vi "test_ImageAssemblerMG090623Binning.vi"() -> ()   [LabVIEW 2010, in "ImageAssemblerMG090623Binning.lvclass"]
uses:
  ImageAssemblerMG090623Binning.lvclass
  main/labview_source/type_definitions/clusters/controls_refs.ctl
  <vilib>/vision/Image Controls.llb/IMAQ Image.ctl
  common/classes/Image/Image/Image.lvclass
  GenericImageAssembler/GenericImageAssembler/trigger_enum.ctl
  ImageAssemblerMG090623Binning.lvclass/ImageAssemblerMG090623Binning.ctl
  GenericImageAssembler/GenericImageAssembler/GenericImageAssembler.lvclass
panel:
  in  "frame rate for sending":dbl[unit]=20.0
  in  "frame rate":dbl[unit]=1.0
  in  "number of images to send":i32=2
  out "loop counter":i32
  in  "send continuously button":bool
  in  "start button":bool
  in  "y resolution":i32=100
  out "input image array":T1[](array[plugin-control])
  in  "stop":bool
  in  "x resolution":i32=100
  in  "number of channels":i32=1 min=1
  in  "send  button":bool
  in  "load button":bool
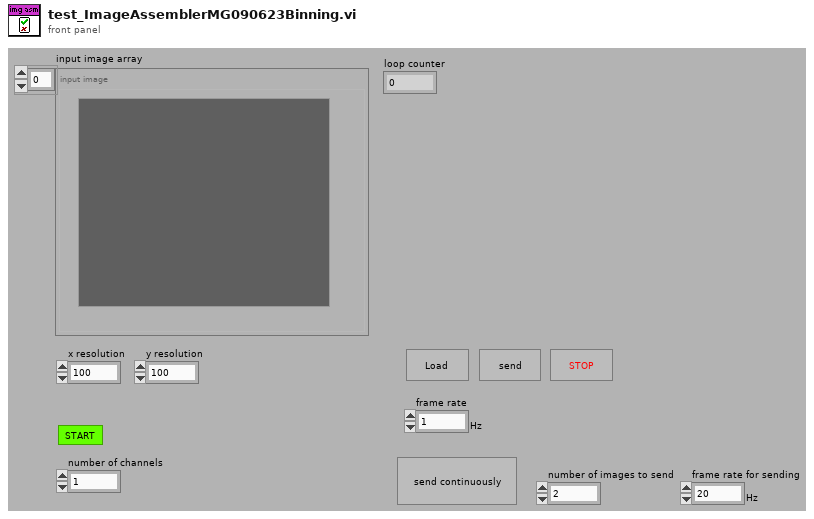
[diagram p1: front panel]
types:
  T1 = typedef "IMAQ Image.ctl" = refnum<image>
  T2 = typedef "Image Type" = u32
  T3 = typedef "controls_refs.ctl" = cluster{"scan start button":refnum<vi>, "tabs":cluster{"main":refnum<vi>, "settings":refnum<vi>}, "subpanels":cluster{"imagingMode":refnum<vi>, "scanHead":refnum<vi>, "display":refnum<vi>, "experimentController":refnum<vi>, "instrument":refnum<vi>, "stage":refnum<vi>, "stimulator":refnum<vi>, "dataCollection":refnum<vi>, "analyser":refnum<vi>, "daq":refnum<vi>, "imageAssembler":refnum<vi>}, "drop-downs":cluster{"run mode":refnum<vi>, "imagingMode":refnum<vi>, "experimentalController":refnum<vi>, "objective":refnum<vi>}, "status lights":cluster{"experimentController":refnum<vi>, "imagingMode":refnum<vi>, "scanHead":refnum<vi>, "daq":refnum<vi>, "imageAssembler":refnum<vi>, "dataCollection":refnum<vi>, "display":refnum<vi>, "analyser":refnum<vi>, "stage":refnum<vi>, "stimulator":refnum<vi>, "instrument":refnum<vi>}, "message":refnum<vi>, "stimulator enabled?":refnum<vi>, "saving":cluster{"data folder path":refnum<vi>, "file base name":refnum<vi>, "notebook":refnum<vi>}, "progress bar":refnum<vi>, "update icon":refnum<vi>, "title":refnum<vi>, "main vi":refnum<vi>, "user":refnum<vi>, "exit_button":refnum<vi>, "CPU usage %":refnum<vi>}
  T4 = typedef "GenericImageAssembler.lvclass/trigger_enum.ctl" = enum16{"NULL", "start", "stop"}
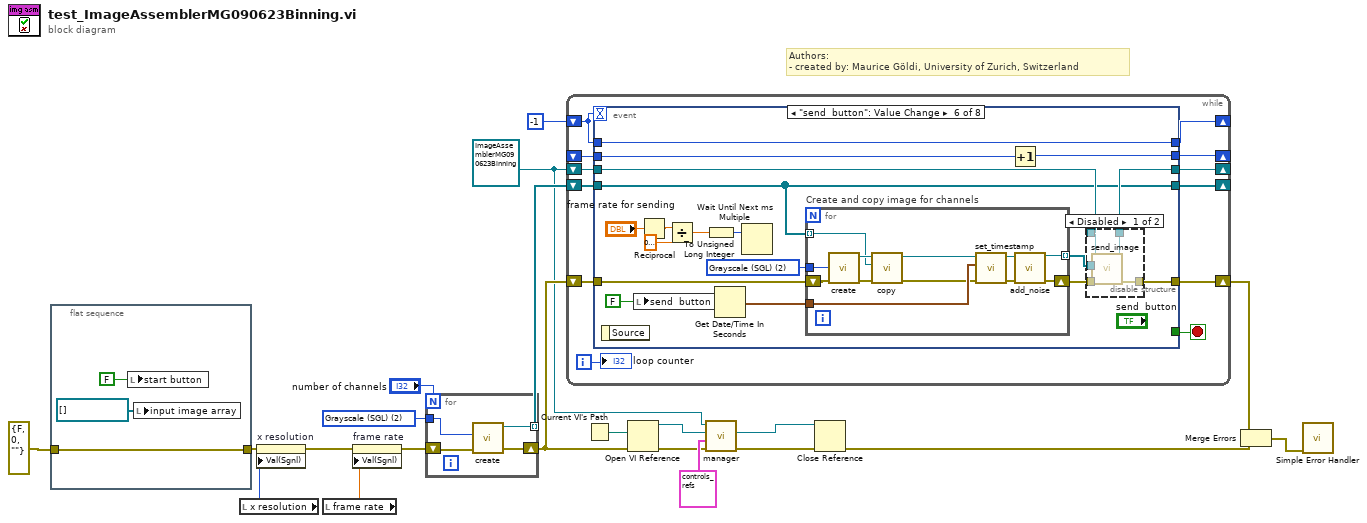
[diagram p0: block diagram]
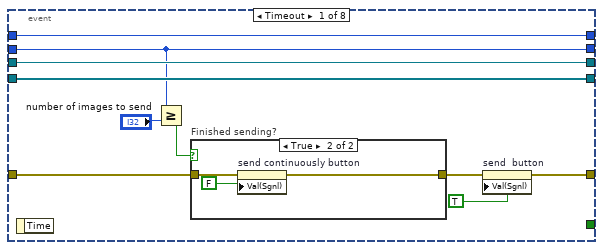
[diagram p2: hidden frame]
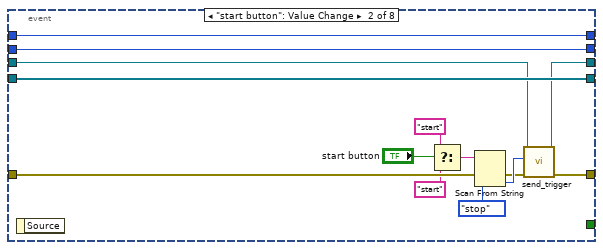
[diagram p4: hidden frame]
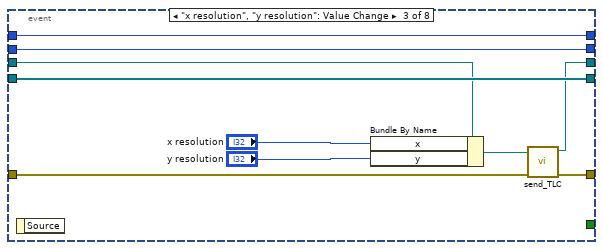
[diagram p5: hidden frame]
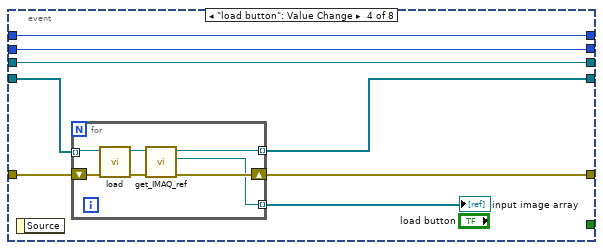
[diagram p6: hidden frame]
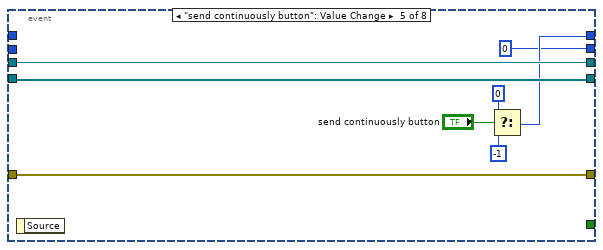
[diagram p7: hidden frame]
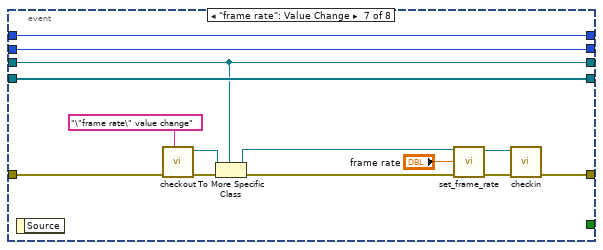
[diagram p9: hidden frame]
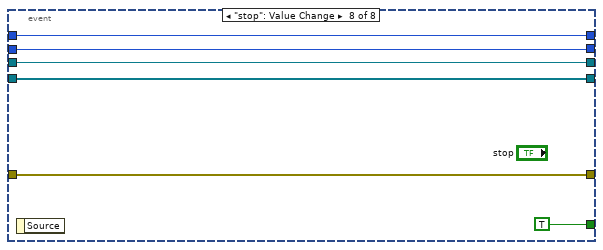
[diagram p10: hidden frame]
diagram:
  w1 = refnum<class "ImageAssemblerMG090623Binning.lvclass"> refnum ("MG090623BinningImageAssembler.lvclass")
  w13 = T2 2 items=["Grayscale (U8)", "Grayscale (I16)", "Grayscale (SGL)", "Complex (CSG)", "RGB (U32)", "HSL (U32)", "RGB (U64)", "Grayscale (U16)"] ("Image Type")
  # "Authors: \n- created by: Maurice Göldi, University of Zurich, Switzerland"
  n1 = flat-sequence {
    tunnel: errorcluster {"status"=FALSE, "code"=0, "source"=""} ("error in (no error)") -> [w24]
    tunnel: [w24] -> w11
    frame #0 {
      n2 = local write "start button"(FALSE ("start button")) -> ()
      n3 = local write "input image array"(T1[] [] ("input image array")) -> ()
    }
  }
  n4 = local read "x resolution"() -> (w14:i32)
  n5 = property on="x resolution" class="DigNum (strict)"(error in=w11, "Val(Sgnl)"=w14) -> (error out=w7:errorcluster)  [unwired: 1 in, 1 out]
  n6 = local read "frame rate"() -> (w6:dbl[unit])
  n7 = property on="frame rate" class="DigNum (strict)"(error in=w7, "Val(Sgnl)"=w6) -> (error out=w5:errorcluster)  [unwired: 1 in, 1 out]
  n8 = for {
    N: "number of channels" -> [_]
    shift-right: [w27] -> w10
    shift-left: w5 -> [w28]
    tunnel: [w26] -> w8 mode=indexing
    tunnel: w13 -> [w25]
    n9 = call "create.vi"("error in (no error)"=w28, "Image Type"=w25) -> ("error out"=w27:errorcluster, "Image out"=w26:refnum<class "Image.lvclass">)  [unwired: 2 in, 6 out]
  }
  n10 = while {
    shift-right: [w34] -> w21
    shift-left: w10 -> [w35]
    shift-right: [w40] -> _
    shift-left: w1 -> [w39]
    shift-right: [w38] -> _
    shift-left: w8 -> [w37]
    shift-right: [w32] -> _
    shift-left: -1 -> [w33]
    shift-right: [w30] -> _
    shift-left: _ -> [w29]
    i -> [w31]
    stop <- w36 stop-if-true
    n11 = event shown="[5] \"send  button\": Value Change" {
      selector: _ -> [_ _ _ _ _ _ _ _]
      dyn-events: _ -> [_ _ _ _ _ _ _ _]
      timeout: w33 -> [_ _ _ _ _ _ _ _]
      tunnel: [w50 w65 w69 w80 w100 w116 w144 w156] -> w40
      tunnel: w39 -> [w50 w66 w74 w80 w100 w117 w144 w156]
      tunnel: [w49 w68 w78 w82 w101 w112 w150 w155] -> w38
      tunnel: w37 -> [w49 w68 w78 w84 w101 w112 w150 w155]
      tunnel: [_ _ _ _ _ _ _ TRUE] -> w36
      tunnel: [w48 w64 w75 w81 w98 w118 w143 w153] -> w34
      tunnel: w35 -> [w43 w59 w76 w85 w98 w114 w139 w153]
      tunnel: w33 -> [w46 w67 w77 w86 _ w119 w149 w152]
      tunnel: [w46 w67 w77 w86 w97 w119 w149 w152] -> w32
      tunnel: [w45 w62 w70 w79 0 w108 w148 w151] -> w30
      tunnel: w29 -> [w45 w62 w70 w79 _ w109 w148 w151]
      event Timeout {
        n12 = event-data() -> ()  [unwired: 2 out]
        n13 = Greater Or Equal?(x=w45, y="number of images to send") -> (x >= y?=w41:bool)
        n14 = case "Finished sending?" shown="True" w41 {
          tunnel: w43 -> [w51 w54]
          tunnel: [w51 w53] -> w42
          frame False {
          }
          frame True {
            n15 = property on="send continuously button" class="Bool (strict)"(error in=w54, "Val(Sgnl)"=FALSE) -> (error out=w53:errorcluster)  [unwired: 1 in, 1 out]
          }
        }
        n16 = property on="send  button" class="Bool (strict)"(error in=w42, "Val(Sgnl)"=TRUE ("Value (Signaling)")) -> (error out=w48:errorcluster)  [unwired: 1 in, 1 out]
      }
      event "start button": Value Change {
        n17 = event-data() -> ()  [unwired: 2 out]
        n18 = Select(t="start" ("input string"), s="start button", f="start" ("input string")) -> (s? t:f=w56:string)
        n19 = Scan From String(input string=w56, error in=w59, default 1=trigger_enum."stop" ("trigger")) -> (error out=w58:errorcluster, output 1=w60:T4)  [unwired: 2 in, 2 out]
        n20 = call-dynamic "send_trigger.vi"("error in (no error)"=w58, "trigger"=w60, "GenericImageAssembler in"=w66) -> ("error out"=w64:errorcluster, "GenericImageAssembler out"=w65:refnum<class "ImageAssemblerMG090623Binning.lvclass">)  [unwired: 7 out]
      }
      event "x resolution", "y resolution": Value Change {
        n21 = event-data() -> ()  [unwired: 2 out]
        n22 = Bundle By Name(cluster=w74, "x"="x resolution", "y"="y resolution") -> (w73:refnum<class "ImageAssemblerMG090623Binning.lvclass">)
        n23 = call-dynamic "send_TLC.vi"("error in (no error)"=w76, "GenericToplevelComponent in"=w73) -> ("error out"=w75:errorcluster, "GenericToplevelComponent out"=w69:refnum<class "ImageAssemblerMG090623Binning.lvclass">)  [unwired: 8 in]
      }
      event "load button": Value Change {
        n24 = event-data() -> ()  [unwired: 2 out]
        n25 = for {
          tunnel: w84 -> [w92] mode=indexing
          tunnel: [w88] -> w82 mode=indexing
          shift-right: [w90] -> w81
          shift-left: w85 -> [w93]
          tunnel: [w87] -> w83 mode=indexing
          n26 = call-dynamic "load.vi"("error in (no error)"=w93, "Image in"=w92) -> ("error out"=w91:errorcluster, "Image out"=w89:refnum<class "Image.lvclass">)  [unwired: 2 in, 6 out]
          n27 = call-dynamic "get_IMAQ_ref.vi"("error in (no error)"=w91, "Image.lvclass in"=w89) -> ("error out"=w90:errorcluster, "Image"=w87:T1, "Image.lvclass out"=w88:refnum<class "Image.lvclass">)  [unwired: 7 out]
        }
        "input image array" <- w83
      }
      event "send continuously button": Value Change {
        n28 = event-data() -> ()  [unwired: 2 out]
        n29 = Select(t=0, s="send continuously button", f=-1) -> (s? t:f=w97:i32)
      }
      event "send  button": Value Change {
        w102 = T2 2 items=["Grayscale (U8)", "Grayscale (I16)", "Grayscale (SGL)", "Complex (CSG)", "RGB (U32)", "HSL (U32)", "RGB (U64)", "Grayscale (U16)"] ("Image Type")
        n30 = event-data() -> ()  [unwired: 2 out]
        n31 = local write "send  button"(FALSE ("send  button")) -> ()
        n32 = Reciprocal(x="frame rate for sending") -> (1/x=w106:dbl[unit])
        n33 = Divide(x=w106, y=dbl[unit] 0.001) -> (x/y=w103:dbl)
        n34 = To Unsigned Long Integer(number=w103) -> (unsigned 32bit integer=w104:u32)
        n35 = Get Date/Time In Seconds() -> (seconds since 1Jan1904=w115:timestamp)
        n36 = Wait Until Next ms Multiple(millisecond multiple=w104) -> ()  [unwired: 1 out]
        n37 = for "Create and copy image for channels" {
          tunnel: w112 -> [w125] mode=indexing
          shift-right: [w132] -> w113
          shift-left: w114 -> [w130]
          tunnel: w115 -> [w136]
          tunnel: [w133] -> w111 mode=indexing
          tunnel: w102 -> [w128]
          n38 = call "create.vi"("error in (no error)"=w130, "Image Type"=w128) -> ("error out"=w131:errorcluster, "Image out"=w126:refnum<class "Image.lvclass">)  [unwired: 2 in, 6 out]
          n39 = call "copy.vi"("error in (no error)"=w131, "image to copy (source)"=w125, "Image in (target)"=w126) -> ("error out"=w129:errorcluster, "Image out"=w127:refnum<class "Image.lvclass">)  [unwired: 7 out]
          n40 = call-dynamic "set_timestamp.vi"("error in (no error)"=w129, "timestamp"=w136, "Image.lvclass in"=w127) -> ("error out"=w135:errorcluster, "Image.lvclass out"=w134:refnum<class "Image.lvclass">)  [unwired: 7 out]
          n41 = call "add_noise.vi"("error in (no error)"=w135, "Image in"=w134) -> ("error out"=w132:errorcluster, "Image out"=w133:refnum<class "Image.lvclass">)  [unwired: 1 in, 7 out]
        }
        n42 = Increment(x=w109) -> (x+1=w108:i32)
        n43 = disable-structure shown="Disabled" {
          disable-tunnel: [w124 _] -> w118
          disable-tunnel: w117 -> [w123 _]
          disable-tunnel: [w122 _] -> w116
          disable-tunnel: w113 -> [w121 _]
          disable-tunnel: w111 -> [w120 _]
          frame Disabled {
            n44 = call-dynamic "send_image.vi"("error in (no error)"=w121, "image (channels)"=w120, "GenericToplevelComponent in"=w123) -> ("error out"=w124:errorcluster, "GenericToplevelComponent out"=w122:refnum<class "ImageAssemblerMG090623Binning.lvclass">)  [unwired: 2 in, 5 out]
          }
          frame Enabled {
          }
        }
      }
      event "frame rate": Value Change {
        n45 = event-data() -> ()  [unwired: 2 out]
        n46 = call "checkout.vi"("locked by?"="\"frame rate\" value change", "error in (no error)"=w139) -> ("error out"=w140:errorcluster, "GenericImageAssembler out"=w138:refnum<class "GenericImageAssembler.lvclass">)  [unwired: 8 out]
        n47 = To More Specific Class(target class=w144, reference=w138, error in=w140) -> (specific class reference=w145:refnum<class "ImageAssemblerMG090623Binning.lvclass">, error out=w147:errorcluster)
        n48 = call-dynamic "set_frame_rate.vi"("error in (no error)"=w147, "frame rate"="frame rate", "MG090623BinningImageAssembler.lvclass in"=w145) -> ("error out"=w142:errorcluster, "MG090623BinningImageAssembler.lvclass out"=w141:refnum<class "ImageAssemblerMG090623Binning.lvclass">)  [unwired: 7 out]
        n49 = call-dynamic "checkin.vi"("error in (no error)"=w142, "GenericImageAssembler in"=w141) -> ("error out"=w143:errorcluster)  [unwired: 8 in, 1 out]
      }
      event "stop": Value Change {
        n50 = event-data() -> ()  [unwired: 2 out]
      }
    }
    "loop counter" <- w31
  }
  n51 = Current VI's Path() -> (path=w17:path)
  n52 = Open VI Reference(vi path=w17, error in (no error)=w10) -> (vi reference=w15:refnum<vi>, error out=w16:errorcluster)  [unwired: 4 out]
  n53 = call-dynamic "manager.vi"("error in (no error)"=w16, "control references"=T3 {"scan start button"=refnum, "tabs"={"main"=refnum, "settings"=refnum}, "subpanels"={"imagingMode"=refnum, "scanHead"=refnum, "display"=refnum, "experimentController"=refnum, "instrument"=refnum, "stage"=refnum, "stimulator"=refnum, "dataCollection"=refnum, "analyser"=refnum, "daq"=refnum, "imageAssembler"=refnum}, "drop-downs"={"run mode"=refnum, "imagingMode"=refnum, "experimentalController"=refnum, "objective"=refnum}, "status lights"={"experimentController"=refnum, "imagingMode"=refnum, "scanHead"=refnum, "daq"=refnum, "imageAssembler"=refnum, "dataCollection"=refnum, "display"=refnum, "analyser"=refnum, "stage"=refnum, "stimulator"=refnum, "instrument"=refnum}, "message"=refnum, "stimulator enabled?"=refnum, "saving"={"data folder path"=refnum, "file base name"=refnum, "notebook"=refnum}, "progress bar"=refnum, "update icon"=refnum, "title"=refnum, "main vi"=refnum, "user"=refnum, "exit_button"=refnum, "CPU usage %"=refnum}, "top-level VI ref in"=w15, "GenericToplevelComponent in"=w1) -> ("error out"=w4:errorcluster, "top-level VI ref out"=w2:refnum<vi>)  [unwired: 5 in, 1 out]
  n54 = Close Reference(reference=w2, error in (no error)=w4) -> (error out=w3:errorcluster)
  n55 = Merge Errors(w21, w3) -> (w20:errorcluster)
  n56 = call <vilib>:"Simple Error Handler.vi"("error in (no error)"=w20) -> ()  [unwired: 1 in, 8 out]
